vi "Gamepad Speed Drive.vi"(7 "Quick Turn":bool, 9 "Turn":dbl, 10 "Speed":dbl) -> (1 "Right Output":dbl, 2 "Left Output":dbl)   [LabVIEW 2011]
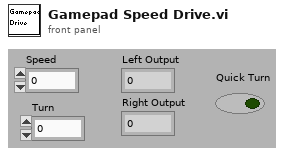
[diagram p1: front panel]
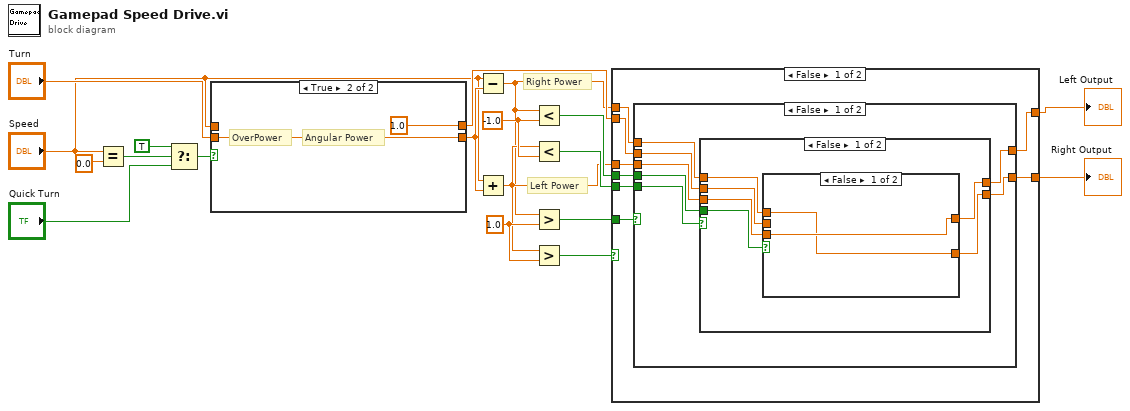
[diagram p0: block diagram]
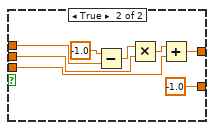
[diagram p2: hidden frame]
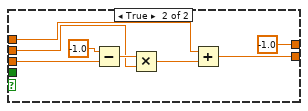
[diagram p3: hidden frame]
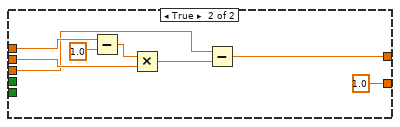
[diagram p4: hidden frame]
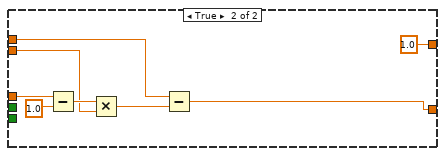
[diagram p5: hidden frame]
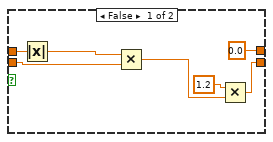
[diagram p6: hidden frame]
diagram:
  w13 = -1.0 ("y")
  w16 = 1.0 ("y")
  # "Right Power"
  # "Left Power"
  n1 = Equal?(x="Speed", y=0.0) -> (x = y?=w4:bool)
  n2 = Select(t=TRUE, s=w4, f="Quick Turn") -> (s? t:f=w3:bool)
  n3 = case shown="True" w3 {
    tunnel: "Turn" -> [w24 w27]
    tunnel: "Speed" -> [w26 _]
    tunnel: [0.0 1.0] -> w10
    tunnel: [w21 w27] -> w18
    frame False {
      n4 = Absolute Value(x=w26) -> (abs(x)=w25:dbl)
      n5 = Multiply(x=w25, y=w24) -> (x*y=w23:dbl)
      n6 = Multiply(x=1.2, y=w23) -> (x*y=w21:dbl)
    }
    frame True {
      # "Angular Power"
      # "OverPower"
    }
  }
  n7 = Subtract(x="Speed", y=w18) -> (x-y=w9:dbl)
  n8 = Add(x="Speed", y=w18) -> (x+y=w11:dbl)
  n9 = Less?(x=w9, y=w13) -> (x < y?=w12:bool)
  n10 = Less?(x=w11, y=w13) -> (x < y?=w14:bool)
  n11 = Greater?(x=w9, y=w16) -> (0:w15:bool)
  n12 = Greater?(x=w11, y=w16) -> (0:w17:bool)
  n13 = case shown="False" w17 {
    tunnel: w15 -> [w36 _]
    tunnel: w14 -> [w35 _]
    tunnel: w12 -> [w34 _]
    tunnel: w11 -> [w30 w83]
    tunnel: w10 -> [w31 w80]
    tunnel: w9 -> [w32 w78]
    tunnel: [w33 w77] -> w7
    tunnel: [w29 1.0] -> w8
    frame False {
      n14 = case shown="False" w36 {
        tunnel: w35 -> [w43 _]
        tunnel: w34 -> [w42 _]
        tunnel: [w38 1.0] -> w33
        tunnel: w32 -> [w39 w71]
        tunnel: w31 -> [w40 w70]
        tunnel: w30 -> [w41 w69]
        tunnel: [w37 w68] -> w29
        frame False {
          n15 = case shown="False" w43 {
            tunnel: w42 -> [w49 _]
            tunnel: w41 -> [w46 w66]
            tunnel: w40 -> [w47 w64]
            tunnel: w39 -> [w48 w62]
            tunnel: [w44 w61] -> w38
            tunnel: [w45 -1.0] -> w37
            frame False {
              n16 = case shown="False" w49 {
                tunnel: w48 -> [w50 w58]
                tunnel: w47 -> [_ w56]
                tunnel: w46 -> [w51 w54]
                tunnel: [w51 w53] -> w45
                tunnel: [w50 -1.0] -> w44
                frame False {
                }
                frame True {
                  n17 = Subtract(x=-1.0, y=w58) -> (x-y=w57:dbl)
                  n18 = Multiply(x=w57, y=w56) -> (x*y=w55:dbl)
                  n19 = Add(x=w55, y=w54) -> (x+y=w53:dbl)
                }
              }
            }
            frame True {
              n20 = Subtract(x=-1.0, y=w66) -> (x-y=w65:dbl)
              n21 = Multiply(x=w65, y=w64) -> (x*y=w63:dbl)
              n22 = Add(x=w62, y=w63) -> (x+y=w61:dbl)
            }
          }
        }
        frame True {
          n23 = Subtract(x=w71, y=1.0) -> (x-y=w74:dbl)
          n24 = Multiply(x=w74, y=w70) -> (x*y=w75:dbl)
          n25 = Subtract(x=w69, y=w75) -> (x-y=w68:dbl)
        }
      }
    }
    frame True {
      n26 = Subtract(x=w83, y=1.0) -> (x-y=w81:dbl)
      n27 = Multiply(x=w81, y=w80) -> (x*y=w79:dbl)
      n28 = Subtract(x=w78, y=w79) -> (x-y=w77:dbl)
    }
  }
  "Left Output" <- w8
  "Right Output" <- w7
